vi "Generate PicoScope 5000a Series Data.vi"(0 "handle in":i16, 1 "Max ADC":i16=32767, 2 "Ch1 Range Index":u16, 3 "Ch2 Range Index":u16, 4 "Actual Sample Interval":dbl, 5 "error in (no error)":errorcluster, 6 "t0":timestamp, 8 "Channel 1 Buff In":refnum<data-value>, 10 "Channel 2 Buff In":refnum<data-value>) -> (7 "next t0":timestamp, 9 "Channel 1 Buff Out":refnum<data-value>, 11 "Channel 2 Buff Out":refnum<data-value>, 14 "handle out":i16, 16 "Graph Data":waveform(dbl)[](array[waveform]), 19 "error out":errorcluster)   [LabVIEW 2016, in "Acquisition.lvlib"]
doc: "Generates sample waveforms according to the signal type in the HW Config input."
uses:
  Acquisition.lvlib
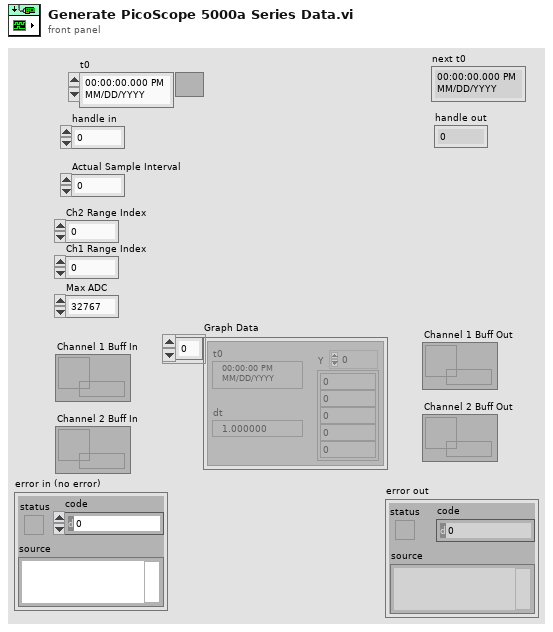
[diagram p1: front panel]
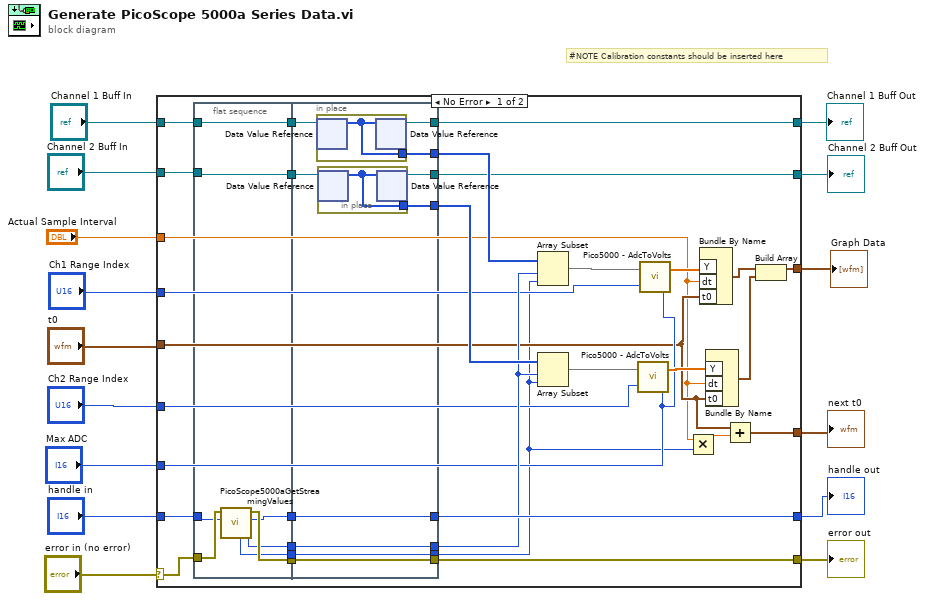
[diagram p0: block diagram]
diagram:
  # "#NOTE Calibration constants should be inserted here"
  n1 = case shown="No Error" "error in (no error)" {
    selector: "error in (no error)" -> [w44 w71]
    tunnel: [w42 w71] -> w14
    tunnel: [w47 _] -> w7
    tunnel: "Channel 1 Buff In" -> [w46 w68]
    tunnel: [w45 w68] -> w12
    tunnel: "handle in" -> [w43 w70]
    tunnel: [w41 w70] -> w10
    tunnel: "Channel 2 Buff In" -> [w40 w69]
    tunnel: [w38 w69] -> w8
    tunnel: "Actual Sample Interval" -> [w24 _]
    tunnel: "Ch1 Range Index" -> [w32 _]
    tunnel: "Max ADC" -> [w27 _]
    tunnel: "Ch2 Range Index" -> [w29 _]
    tunnel: "t0" -> [w25 _]
    tunnel: [w22 _] -> w1
    frame No Error {
      n2 = flat-sequence {
        tunnel: w46 -> [w49]
        tunnel: w44 -> [w55]
        tunnel: w43 -> [w54]
        tunnel: w40 -> [w48]
        tunnel: [w49] -> w21
        tunnel: [w53] -> w20
        tunnel: [w52] -> w19
        tunnel: [w48] -> w18
        tunnel: [w51] -> w17
        tunnel: [w50] -> w16
        tunnel: [w62] -> w23
        tunnel: [w63] -> w36
        tunnel: [w56] -> w37
        tunnel: [w59] -> w38
        tunnel: [w57] -> w39
        tunnel: [w64] -> w41
        tunnel: [w65] -> w42
        tunnel: [w58] -> w45
        tunnel: w21 -> [w61]
        tunnel: w20 -> [w65]
        tunnel: w19 -> [w64]
        tunnel: w18 -> [w60]
        tunnel: w17 -> [w63]
        tunnel: w16 -> [w62]
        frame #0 {
          n3 = call "PicoScope5000aGetStreamingValues.vi"("handle in"=w54, "error in"=w55) -> ("Start Index in Driver Buffer"=w51:u32, "handle out"=w52:i16, "error out"=w53:errorcluster, "Number of Samples"=w50:u32)  [unwired: 4 in, 2 out]
        }
        frame #1 {
          n4 = in-place {
            in-place-border: [w67] -> w57
            n5 = in-place-dvr #1(w61) -> (w67:i16[])  [unwired: 1 out]
            n6 = in-place-dvr #1(w67) -> (w58:refnum<data-value>)  [unwired: 1 out]
          }
          n7 = in-place {
            in-place-border: [w66] -> w56
            n8 = in-place-dvr #2(w60) -> (w66:i16[])  [unwired: 1 out]
            n9 = in-place-dvr #2(w66) -> (w59:refnum<data-value>)  [unwired: 1 out]
          }
        }
      }
      n10 = Array Subset(array=w39, index=w36, length=w23) -> (w34:i16[])
      n11 = Array Subset(array=w37, index=w36, length=w23) -> (w30:i16[])
      n12 = call "Pico5000 - AdcToVolts.vi"("Max ADC"=w27, "Range Index"=w29, "Data"=w30) -> ("Data (Volts)"=w31:dbl[])
      n13 = call "Pico5000 - AdcToVolts.vi"("Max ADC"=w27, "Range Index"=w32, "Data"=w34) -> ("Data (Volts)"=w33:dbl[])
      n14 = Multiply(x=w24, y=w23) -> (x*y=w26:dbl)
      n15 = Bundle By Name("Y"=w33, "dt"=w24, "t0"=w25) -> (w35:waveform(dbl))  [unwired: 1 in]
      n16 = Bundle By Name("Y"=w31, "dt"=w24, "t0"=w25) -> (w28:waveform(dbl))  [unwired: 1 in]
      n17 = Add(x=w25, y=w26) -> (x+y=w22:timestamp)
      n18 = Build Array(w35, w28) -> (w47:waveform(dbl)[])
    }
    frame Error {
    }
  }
  "error out" <- w14
  "Graph Data" <- w7
  "Channel 1 Buff Out" <- w12
  "handle out" <- w10
  "Channel 2 Buff Out" <- w8
  "next t0" <- w1
